vi "Invert Greyscale Image In-Place.vi"(8 "error in (no error)":errorcluster, 11 "Greyscale Image to Invert in Place in":T1) -> (0 "error out":errorcluster, 3 "Greyscale Image":T1)   [LabVIEW 2020, in "image.lvlib"]
doc: "Invert the Pixels in the Greyscale Image in-place.\n\nThis function is useful when inverting a Greyscale Image which represents a mask."
uses:
  image.lvlib
  Greyscale Image.ctl
  common/common.lvlib
  common/bin/gartoolkit_32-1.dll
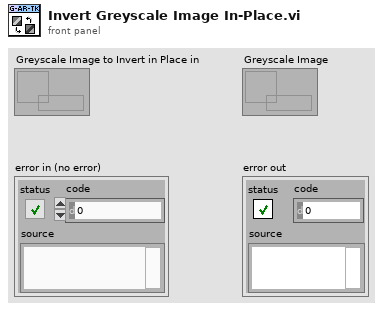
[diagram p1: front panel]
types:
  T1 = typedef "image.lvlib/Greyscale Image.ctl" = refnum<data-value>
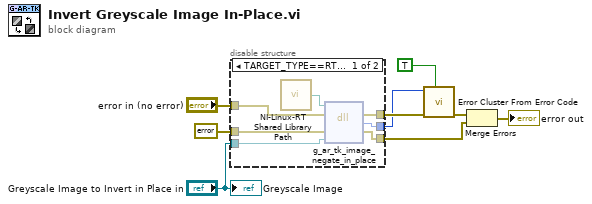
[diagram p0: block diagram]
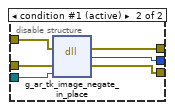
[diagram p2: hidden frame]
diagram:
  n1 = disable-structure shown="TARGET_TYPE==RT&&OS==Linux" {
    disable-tunnel: "error in (no error)" -> [w16 w22]
    disable-tunnel: errorcluster {"status"=FALSE, "code"=0, "source"=""} ("error constant") -> [w15 w21]
    disable-tunnel: "Greyscale Image to Invert in Place in" -> [w14 w20]
    disable-tunnel: [w13 w19] -> w4
    disable-tunnel: [w12 w18] -> w3
    disable-tunnel: [w11 w17] -> w2
    frame condition #0 {
      n2 = call "NI-Linux-RT Shared Library Path.vi"() -> ("Path"=w10:path)
      n3 = dll-call lib="?" fn="g_ar_tk_image_negate_in_place" ("g_ar_toolkit.*.*:g_ar_tk_image_negate")(path in=w10, error in=w16, "error_cluster"=w15, "EDVR image"=w14) -> (error out=w13:errorcluster, w12:i32, "error_cluster"=w11:errorcluster)  [unwired: 2 in, 1 out]
    }
    frame condition #1 (active) {
      n4 = dll-call lib="C:/serenial/lib/g-augmented-reality-toolkit/LabVIEW/common/bin/gartoolkit_*-1.*" fn="g_ar_tk_image_negate_in_place" ("g_ar_toolkit.*.*:g_ar_tk_image_negate")(error in=w22, "error_cluster"=w21, "EDVR image"=w20) -> (error out=w19:errorcluster, w18:i32, "error_cluster"=w17:errorcluster)  [unwired: 3 in, 1 out]
    }
  }
  n5 = call <vilib>:"Error Cluster From Error Code.vi"("show call chain? (False)"=TRUE, "error in (no error)"=w4, "error code (0)"=w3) -> ("error out"=w8:errorcluster)  [unwired: 6 in]
  n6 = Merge Errors(w8, w2) -> (→"error out":errorcluster)
  "Greyscale Image" <- "Greyscale Image to Invert in Place in"
